vi "BRig_dataLC_Cue2_PostR_Count_l1.vi"() -> (2 "output_Cue2_PostR_Count":i32)   [LabVIEW 2014]
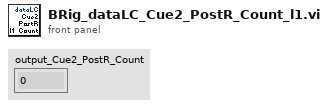
[diagram p1: front panel]
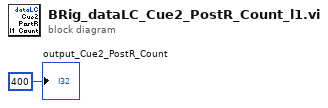
[diagram p0: block diagram]
diagram:
  "output_Cue2_PostR_Count" <- 400 ("output_iBlock")
